vi "Read basicType.vi"(8 "error in (no error)":errorcluster, 11 "Array in":refnum<class "Array.lvclass">) -> (0 "error out":errorcluster, 2 "Primitive.lvclass":refnum<class "Primitive.lvclass">, 3 "Array out":refnum<class "Array.lvclass">)   [LabVIEW 2018, in "Array.lvclass"]
uses:
  Array.lvclass
  Primitive/Primitive.lvclass
  Array.lvclass/Array.ctl
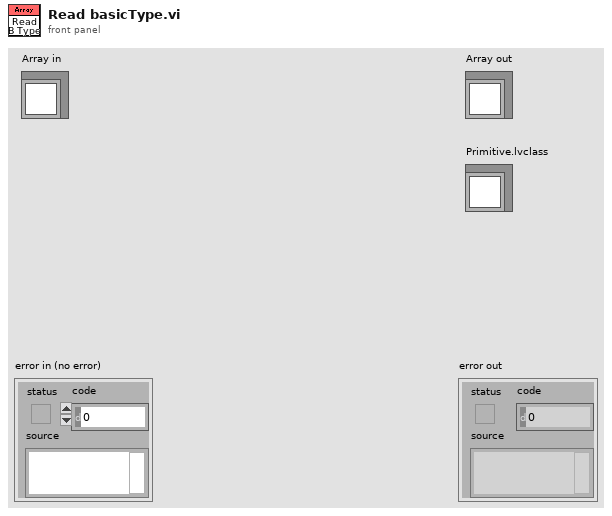
[diagram p1: front panel]
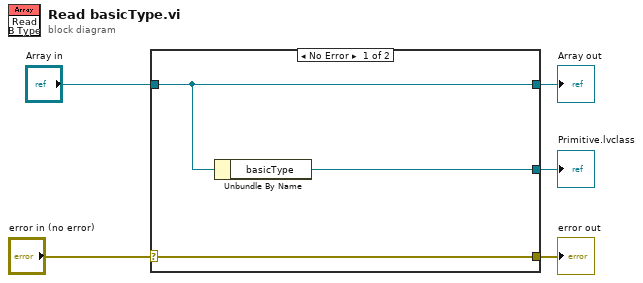
[diagram p0: block diagram]
diagram:
  n1 = case shown="No Error" "error in (no error)" {
    selector: "error in (no error)" -> [w8 w9]
    tunnel: [w8 w9] -> w4
    tunnel: [w7 w10] -> w2
    tunnel: "Array in" -> [w7 w10]
    tunnel: [w6 _] -> w1
    frame No Error {
      n2 = Unbundle By Name(w7) -> ("basicType"=w6:refnum<class "Primitive.lvclass">)
    }
    frame Error {
    }
  }
  "error out" <- w4
  "Array out" <- w2
  "Primitive.lvclass" <- w1
